vi "toBooleanScalar.vi"(2 "value_in":u8[](array[numeric]), 3 "dim_y":i32, 4 "dim_x":i32) -> (0 "setpoint":bool=TRUE, 1 "value_out":bool=TRUE)   [LabVIEW 2014, in "tango.lvlib"]
uses:
  tango.lvlib
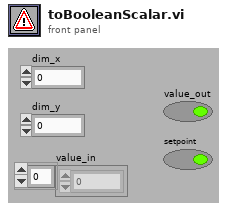
[diagram p1: front panel]
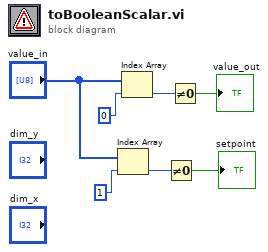
[diagram p0: block diagram]
diagram:
  n1 = Index Array(array="value_in", index=1 ("indice")) -> (element=w3:u8)
  n2 = Index Array(array="value_in", index=0 ("indice")) -> (element=w6:u8)
  n3 = Not Equal To 0?(x=w3) -> (x != 0?=→"setpoint":bool)
  n4 = Not Equal To 0?(x=w6) -> (x != 0?=→"value_out":bool)
